vi "_save_csv_ELTA_EIRP_pdet_power.vi"(7 "delimiter (\\t)":string="SingleCh_", 11 "Data":dbl[][](array[numeric])) -> (3 "FileName":string)   [LabVIEW 2023]
uses:
  <vilib>/Utility/file.llb/Write Delimited Spreadsheet (string).vi
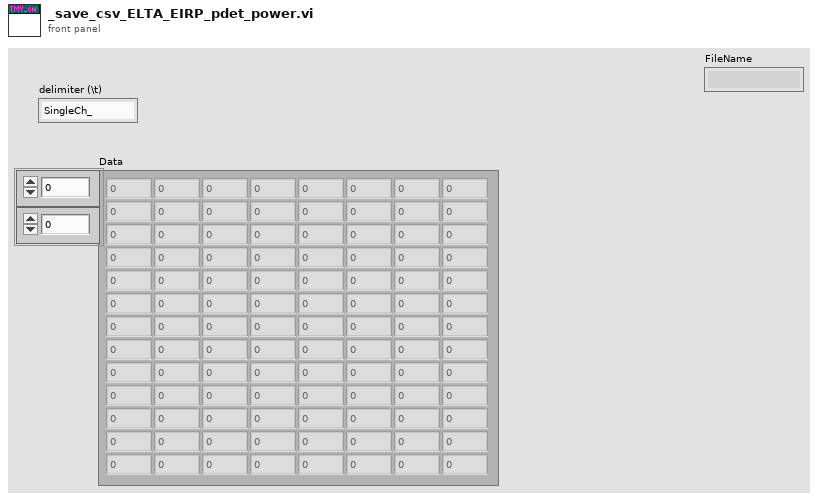
[diagram p1: front panel]
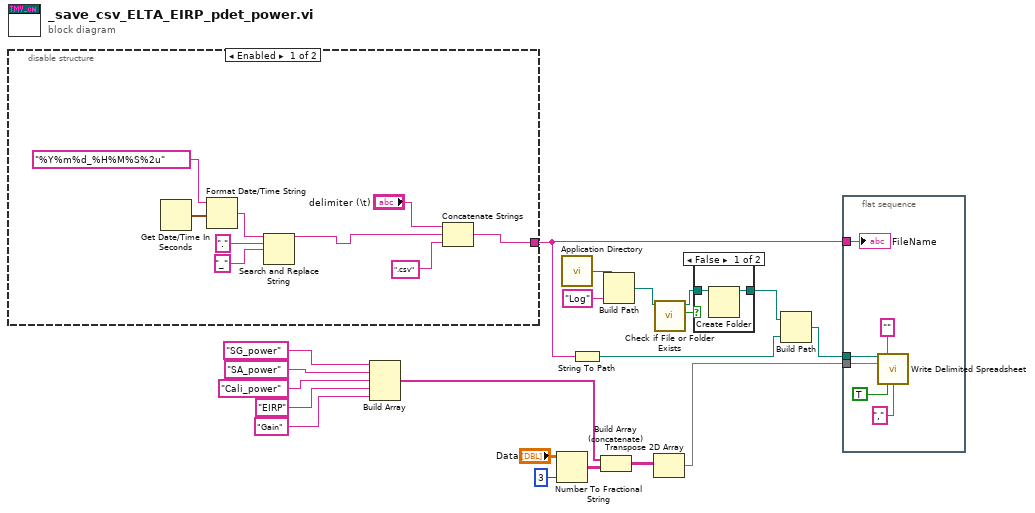
[diagram p0: block diagram]
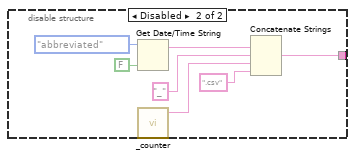
[diagram p3: hidden frame]
diagram:
  n1 = disable-structure shown="Enabled" {
    disable-tunnel: [w28 w30] -> w17
    frame Enabled {
      n2 = Get Date/Time In Seconds() -> (seconds since 1Jan1904=w26:timestamp)
      n3 = Format Date/Time String(time format string (%c)="%Y%m%d_%H%M%S%2u", seconds (now)=w26) -> (date/time string=w24:string)  [unwired: 1 in]
      n4 = Search and Replace String(input string=w24, search string=".", replace string="_") -> (result string=w21:string)  [unwired: 5 in, 3 out]
      n5 = Concatenate Strings("delimiter (\\t)", w21, ".csv" ("delimiter (\\t)")) -> (w28:string)
    }
    frame Disabled {
      n6 = Get Date/Time String(date format (0)=enum16{"short", "long", "abbreviated"}."abbreviated", want seconds? (F)=FALSE) -> (date string=w37:string)  [unwired: 1 in, 1 out]
      n7 = call "_counter.vi"() -> ("out_count"=w31:string)  [unwired: 5 in]
      n8 = Concatenate Strings(w37, "_" ("delimiter (\\t)"), w31, ".csv" ("delimiter (\\t)")) -> (w30:string, w32:string)
    }
  }
  n9 = Build Array("SG_power", "SA_power", "Cali_power", "EIRP", "Gain") -> (w6:string[])
  n10 = Number To Fractional String(number="Data", precision (6)=i16 3) -> (F-format string=w7:string[][])  [unwired: 2 in]
  n11 = call <vilib>:"Application Directory.vi"() -> ("Application Directory"=w16:path)
  n12 = String To Path(string=w17) -> (path=w19:path)
  n13 = Build Array (concatenate)(w6, w7) -> (w5:string[][])
  n14 = Build Path(base path=w16, name or relative path="Log") -> (appended path=w13:path)
  n15 = Transpose 2D Array(2D array=w5) -> (transposed array=w4:string[][])
  n16 = call <vilib>:"Check if File or Folder Exists.vi"("path"=w13) -> ("file or folder exists?"=w15:bool, "dup path"=w14:path)  [unwired: 8 in, 1 out]
  n17 = case shown="False" w15 {
    tunnel: w14 -> [w39 w40]
    tunnel: [w38 w40] -> w12
    frame False {
      n18 = Create Folder(path (use dialog)=w39) -> (created path=w38:path)  [unwired: 2 in, 2 out]
    }
    frame True {
    }
  }
  n19 = Build Path(base path=w12, name or relative path=w19) -> (appended path=w18:path)
  n20 = flat-sequence {
    tunnel: w18 -> [w45]
    tunnel: w17 -> [w43]
    tunnel: w4 -> [w41]
    frame #0 {
      n21 = call-poly <vilib>:"Write Delimited Spreadsheet.vi"("file path (dialog if empty)"=w45, "format (%s)"="" ("format (%.3f)"), "2D data"=w41, "transpose? (no:F)"=TRUE, "delimiter (\\t)"="," ("delimiter (\\t)")) -> ()  [unwired: 9 in, 2 out]
      "FileName" <- w43
    }
  }
